vi "display report.vi"(8 "error in":errorcluster, 11 "data to display":string) -> (0 "error out":errorcluster)   [LabVIEW 2025, in "CEF.lvlib" / "CEF_serializable node.lvclass"]
doc: "Copyright 2017 National Instruments Corporation\n\nLicensed under the Apache License, Version 2.0 (the \"License\"); you may not use this file except in compliance with the License. You may obtain a copy of the License at http://www.apache.org/licenses/LICENSE-2.0\nUnless required by applicable law or agreed to in writing, software distributed under the License is distributed on an \"AS IS\" BASIS, WITHOUT WARRANTIES OR CONDITIONS OF ANY KIND, either express or implied. See the License for the specific language governing permissions and limitations under the License."
uses:
  CEF_serializable node.lvclass
panel:
  in  "OK":bool
  out "report info":string
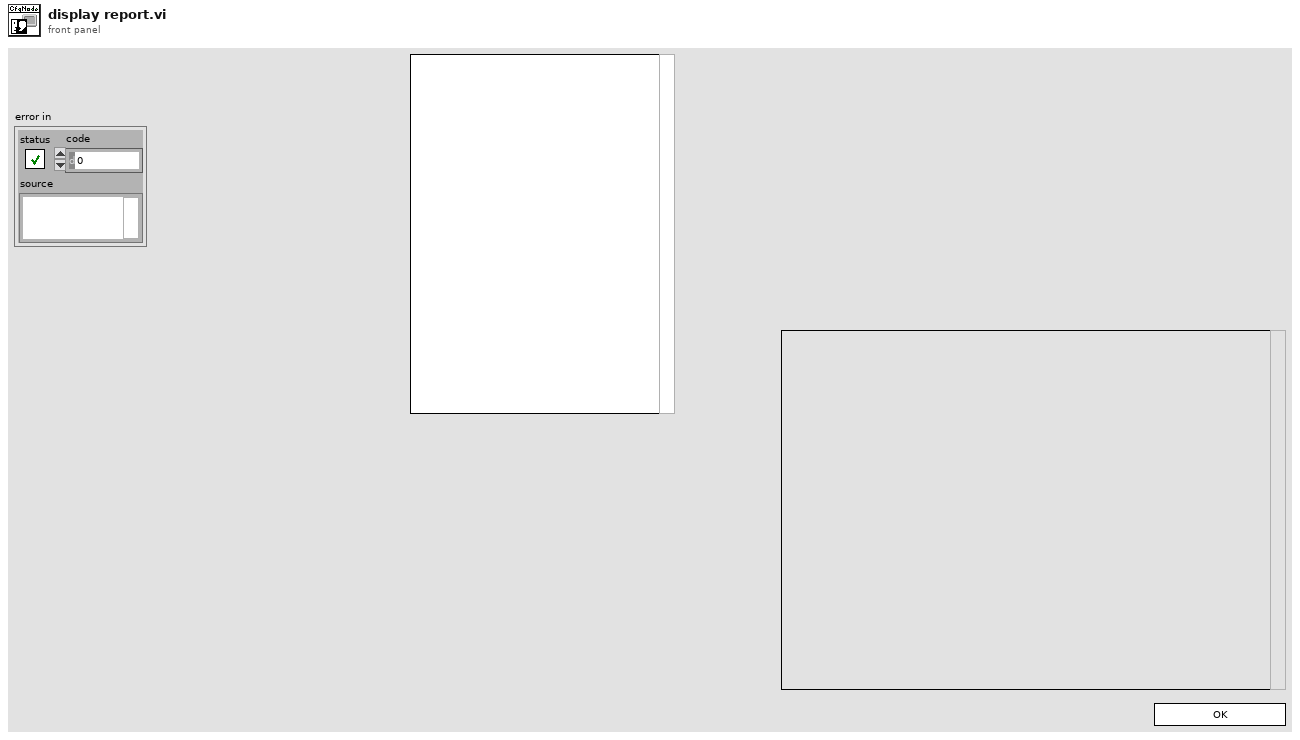
[diagram p1: front panel]
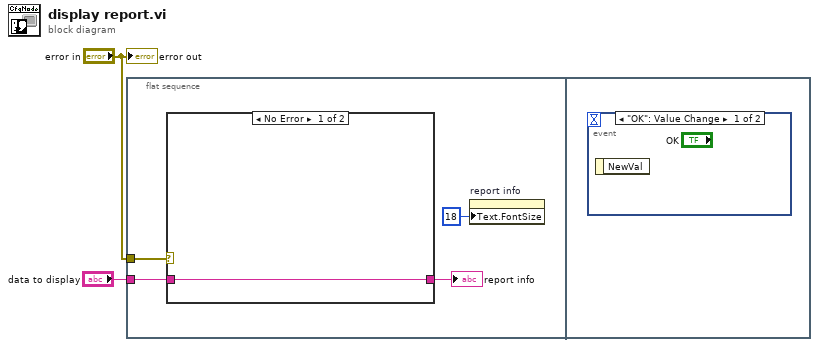
[diagram p0: block diagram]
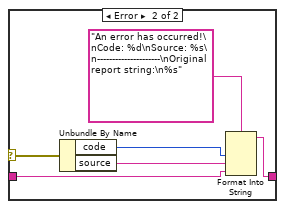
[diagram p2: hidden frame]
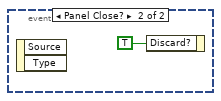
[diagram p3: hidden frame]
diagram:
  n1 = flat-sequence {
    tunnel: "error in" -> [w6]
    tunnel: "data to display" -> [w5]
    frame #0 {
      n2 = case shown="No Error" w6 {
        selector: w6 -> [_ w10]
        tunnel: w5 -> [w7 w11]
        tunnel: [w7 w13] -> w4
        frame No Error {
        }
        frame Error {
          n3 = Unbundle By Name(w10) -> ("code"=w9:i32, "source"=w8:string)
          n4 = Format Into String(format string="An error has occurred!\nCode: %d\nSource: %s\n---------------------\nOriginal report string:\n%s", w9, w8, w11) -> (resulting string=w13:string)  [unwired: 2 in, 1 out]
        }
      }
      "report info" <- w4
      n5 = property on="report info" class="Str"("Text.FontSize"=u32 18 ("Text.Font:Size")) -> ()  [unwired: 2 in, 2 out]
    }
    frame #1 {
      n6 = event shown="[0] \"OK\": Value Change" {
        selector: _ -> [_ _]
        dyn-events: _ -> [_ _]
        timeout: _ -> [_ _]
        event "OK": Value Change {
          n7 = event-data() -> ()  [unwired: 1 in, 1 out]
        }
        event Panel Close? {
          n8 = event-data() -> ()  [unwired: 1 in, 2 out]
          n9 = event-data("Discard?"=TRUE) -> ()  [unwired: 1 in, 1 out]
        }
      }
    }
  }
  "error out" <- "error in"
